vi "Window Position Selector.vi"   [LabVIEW 2020, in "Panel.lvlib"]
doc: "Polymorphic VI to select an appropriate constructor for a window positioner.\n\n----\nPlease see the following web address for additional documentation and tutorial information:\nhttp://www.mooregoodideas.com/mgi-panel-manager/\n\nAuthor: Derek Trepanier\n\nCopyright (c) 2018, Moore Good Ideas, Inc.\n\nAll rights reserved.\n\nRedistribution and use in source and binary forms, with or without modification, are permitted provided that the following conditions are met:\n\n * Redistributions of source code must retain the above copyright notice, this list of conditions and the following disclaimer.\n * Redistributions in binary form must reproduce the above copyright notice, this list of conditions and the following disclaimer in the documentation and/or other materials provided with the distribution.\n * Neither the name of Moore Good Ideas, Inc. nor the names of its contributors may be used to endorse or promote products derived from this software without specific prior written permission.\n\nTHIS SOFTWARE IS PROVIDED BY THE COPYRIGHT HOLDERS AND CONTRIBUTORS \"AS IS\" AND ANY EXPRESS OR IMPLIED WARRANTIES, INCLUDING, BUT NOT LIMITED TO, THE IMPLIED WARRANTIES OF MERCHANTABILITY AND FITNESS FOR A PARTICULAR PURPOSE ARE DISCLAIMED. IN NO EVENT SHALL THE COPYRIGHT OWNER OR CONTRIBUTORS BE LIABLE FOR ANY DIRECT, INDIRECT, INCIDENTAL, SPECIAL, EXEMPLARY, OR CONSEQUENTIAL DAMAGES (INCLUDING, BUT NOT LIMITED TO, PROCUREMENT OF SUBSTITUTE GOODS OR SERVICES; LOSS OF USE, DATA, OR PROFITS; OR BUSINESS INTERRUPTION) HOWEVER CAUSED AND ON ANY THEORY OF LIABILITY, WHETHER IN CONTRACT, STRICT LIABILITY, OR TORT (INCLUDING NEGLIGENCE OR OTHERWISE) ARISING IN ANY WAY OUT OF THE USE OF THIS SOFTWARE, EVEN IF ADVISED OF THE POSSIBILITY OF SUCH DAMAGE."
uses:
  <vilib>/MGI/Panel Manager/Panel/Panel.lvlib
  <vilib>/MGI/Panel Manager/Panel/Window Position/Reference Position/Ref Top Level/Ref Top Level.lvclass
  <vilib>/MGI/Panel Manager/Panel/Window Position/Reference Position/Ref VI/Ref VI.lvclass
  <vilib>/MGI/Panel Manager/Panel/Window Position/Reference Position/Ref Ctrl/Ref Ctrl.lvclass
  <vilib>/MGI/Panel Manager/Panel/Window Position/Maximize/Maximize.lvclass
  <vilib>/MGI/Panel Manager/Panel/Window Position/Reference Position/Ref Display/Ref Display.lvclass
  <vilib>/MGI/Panel Manager/Panel/Window Position/Persistent Position/Persistent Position.lvclass
  <vilib>/MGI/Panel Manager/Panel/Window Position/Reference Position/Ref Rectangle/Ref Rectangle.lvclass
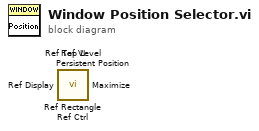
[diagram p0: block diagram]
diagram:
  n1 = call <vilib>:"Ref Rectangle.vi"() -> ()  [unwired: 10 in, 2 out]
  n2 = call <vilib>:"Persistent Position.vi"() -> ()  [unwired: 10 in, 2 out]
  n3 = call <vilib>:"Ref Display.vi"() -> ()  [unwired: 10 in, 2 out]
  n4 = call <vilib>:"Maximize.vi"() -> ()  [unwired: 10 in, 2 out]
  n5 = call <vilib>:"Ref Ctrl.vi"() -> ()  [unwired: 10 in, 2 out]
  n6 = call <vilib>:"Ref VI.vi"() -> ()  [unwired: 10 in, 2 out]
  n7 = call <vilib>:"Ref Top Level.vi"() -> ()  [unwired: 10 in, 2 out]
